vi "Obtain Doc Title.vi"(8 "error in (no error)":errorcluster, 11 "LV RT in":refnum<class "LV RT.lvclass">) -> (0 "error out":errorcluster, 3 "LV RT out":refnum<class "LV RT.lvclass">)   [LabVIEW 2019, in "LV RT.lvclass"]
uses:
  LV RT.lvclass
  D:/Namratha/MDI/LabVIEW-MDI-develop_LV2019/source code/Document/LV Doc/LV Doc.lvclass
  D:/Namratha/MDI/LabVIEW-MDI-develop_LV2019/source code/Document/Document base/Document.lvclass
  LV Doc.lvclass/LV Doc.ctl
  Document base/Document.lvclass/Document.ctl
  property/Read VI Reference.vi
  Document base/property/Write Doc Title.vi
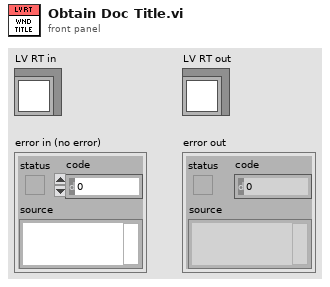
[diagram p1: front panel]
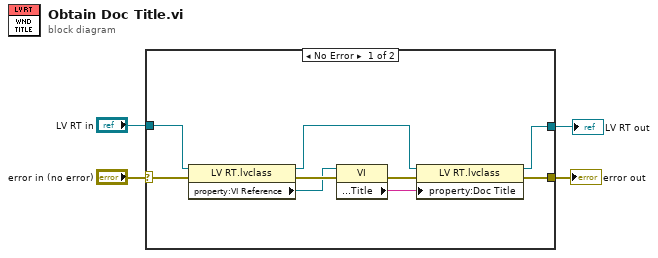
[diagram p0: block diagram]
diagram:
  n1 = case shown="No Error" "error in (no error)" {
    selector: "error in (no error)" -> [w13 w15]
    tunnel: [w5 w15] -> w3
    tunnel: "LV RT in" -> [w12 w14]
    tunnel: [w8 w14] -> w1
    frame No Error {
      n2 = property class="LV RT.lvclass"(reference=w12, error in=w13) -> (reference out=w9:refnum<class "LV RT.lvclass">, error out=w11:errorcluster, "property:VI Reference"=w10:refnum<vi>)
      n3 = property class="VI"(reference=w10, error in=w11) -> (error out=w7:errorcluster, "Front Panel.Title"=w6:string)  [unwired: 1 out]
      n4 = property class="LV RT.lvclass"(reference=w9, error in=w7, "property:Doc Title"=w6) -> (reference out=w8:refnum<class "LV RT.lvclass">, error out=w5:errorcluster)
    }
    frame Error {
    }
  }
  "error out" <- w3
  "LV RT out" <- w1
